vi "distribute_setpoints.vi"(8 "setpoints":dbl[](array[numeric]), 10 "upper layer grid info":T1) -> (2 "references":T2)   [LabVIEW 2021]
uses:
  controls/references.ctl
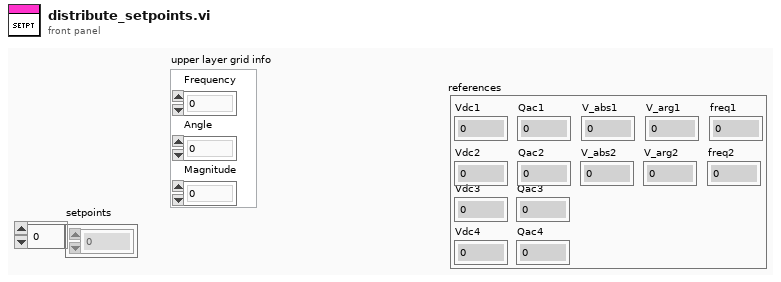
[diagram p1: front panel]
types:
  T1 = cluster{"Frequency":dbl, "Angle":dbl, "Magnitude":dbl}
  T2 = typedef "references.ctl" = cluster{"Vdc1":dbl, "Vdc2":dbl, "Qac2":dbl, "Vdc3":dbl, "Qac3":dbl, "Vdc4":dbl, "Qac4":dbl, "Qac1":dbl, "V_arg2":dbl, "V_abs2":dbl, "V_abs1":dbl, "V_arg1":dbl, "freq1":dbl, "freq2":dbl}
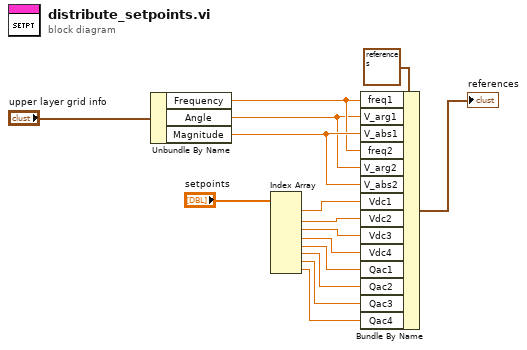
[diagram p0: block diagram]
diagram:
  n1 = Unbundle By Name("upper layer grid info") -> ("Frequency"=w2:dbl, "Angle"=w1:dbl, "Magnitude"=w3:dbl)
  n2 = Index Array(array="setpoints") -> (element #1=w13:dbl, element #2=w11:dbl, element #3=w10:dbl, element #4=w9:dbl, element #5=w8:dbl, element #6=w7:dbl, element #7=w6:dbl, element #8=w5:dbl)  [unwired: 8 in]
  n3 = Bundle By Name(cluster=T2 {"Vdc1"=0.0, "Vdc2"=0.0, "Qac2"=0.0, "Vdc3"=0.0, "Qac3"=0.0, "Vdc4"=0.0, "Qac4"=0.0, "Qac1"=0.0, "V_arg2"=0.0, "V_abs2"=0.0, "V_abs1"=0.0, "V_arg1"=0.0, "freq1"=0.0, "freq2"=0.0} ("references 2"), "freq1"=w2, "V_arg1"=w1, "V_abs1"=w3, "freq2"=w2, "V_arg2"=w1, "V_abs2"=w3, "Vdc1"=w13, "Vdc2"=w11, "Vdc3"=w10, "Vdc4"=w9, "Qac1"=w8, "Qac2"=w7, "Qac3"=w6, "Qac4"=w5) -> (→"references":T2)
